vi "Boolean to Number.vi"() -> ()   [LabVIEW 2020]
panel:
  out "Bin Number":u32 format="%.0b"
  out "Bit 8":bool
  out "Bit 7":bool
  out "Bit 6":bool
  out "Bit 5":bool
  out "Bit 4":bool
  out "Bit 3":bool
  out "Bit 2":bool
  out "Bit 1":bool
  in  "Dec Number":u32
  out "Dec Number":u32
  in  "Bit 8":bool
  in  "Bit 7":bool
  in  "Bit 6":bool
  in  "Bit 5":bool
  in  "Bit 4":bool
  in  "Bit 3":bool
  in  "Bit 2":bool
  in  "Bit 1":bool
  # "Decimal Value"
  # "128"
  # "64"
  # "32"
  # "16"
  # "8"
  # "4"
  # "2"
  # "1"
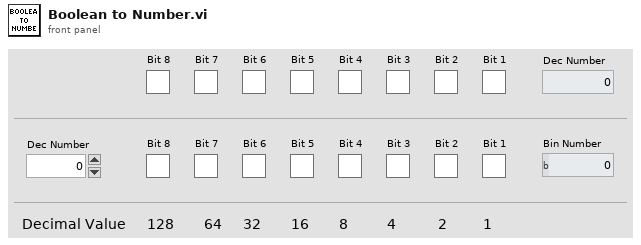
[diagram p1: front panel]
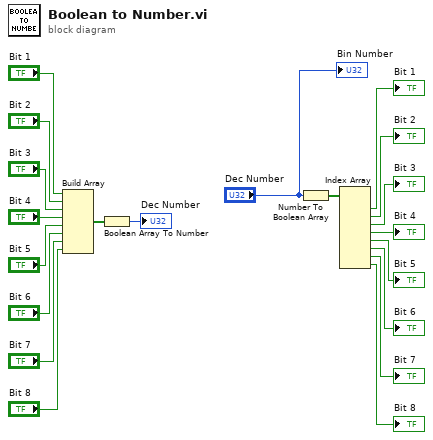
[diagram p0: block diagram]
diagram:
  n1 = Build Array("Bit 1", "Bit 2", "Bit 3", "Bit 4", "Bit 5", "Bit 6", "Bit 7", "Bit 8") -> (w12:bool[])
  n2 = Boolean Array To Number(Boolean array=w12) -> (number=→"Dec Number":u32)
  n3 = Number To Boolean Array(number="Dec Number") -> (Boolean array=w10:bool[])
  n4 = Index Array(array=w10) -> (element #1=→"Bit 1":bool, element #2=→"Bit 2":bool, element #3=→"Bit 3":bool, element #4=→"Bit 4":bool, element #5=→"Bit 5":bool, element #6=→"Bit 6":bool, element #7=→"Bit 7":bool, element #8=→"Bit 8":bool)  [unwired: 8 in]
  "Bin Number" <- "Dec Number"
